vi "myRIO_BRig_RT_dataExp_laser1_duration.vi"() -> (2 "output_laser1_duration":i32)   [LabVIEW 2014]
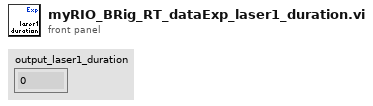
[diagram p1: front panel]
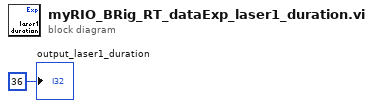
[diagram p0: block diagram]
diagram:
  "output_laser1_duration" <- 36 ("output_iBlock")
